vi "Read Dataset and All Attributes (Variant).vi"(4 "Data":variant, 8 "error in (no error)":errorcluster, 10 "Dataset Path":string, 11 "HDF5 Ref":T1) -> (0 "error out":errorcluster, 1 "Data out":variant, 3 "HDF5 Ref out":T1, 5 "Attribute Values":variant[](array[variant]), 7 "Attribute Names":string[](array[string]))   [LabVIEW 2017]
doc: "Reads a dataset and some or all of its attributes."
uses:
  <vilib>/UPVI/lvhdf5/library.llb/HDF5 Ref.ctl
panel:
  # "LVHDF5 Toolkit\nCopyright (c) 2005-2013 by Jason D. Sommerville\nCopyright (c) 2014 by UPVI, LLC.\n\nThis use and distribution of this file is governed by the terms found in \nLICENSE.txt distributed with this toolkit and installed at\n <user.lib>\\_lvhdf5\\LICENSE.txt"
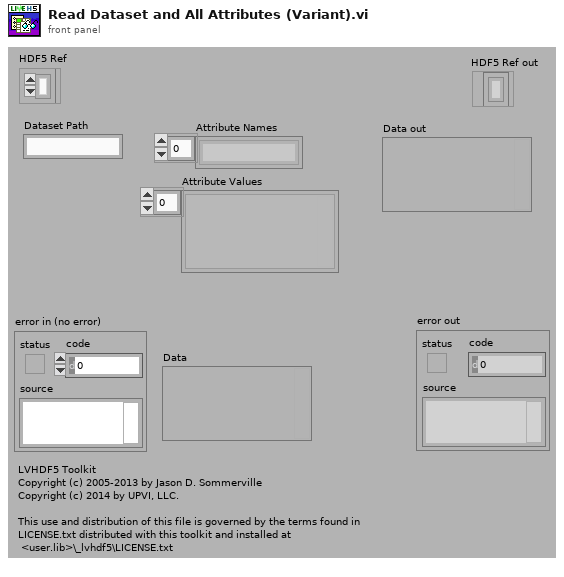
[diagram p1: front panel]
types:
  T1 = typedef "HDF5 Ref.ctl" = refnum<k1>
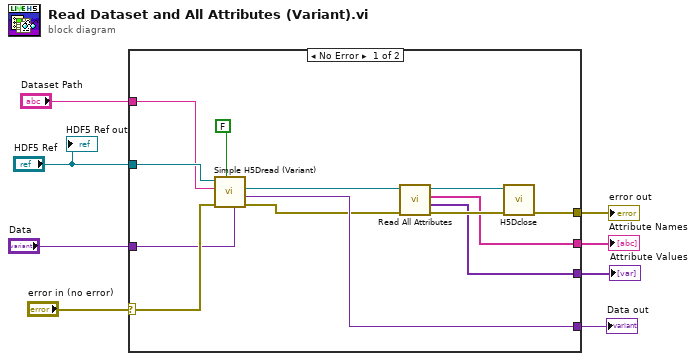
[diagram p0: block diagram]
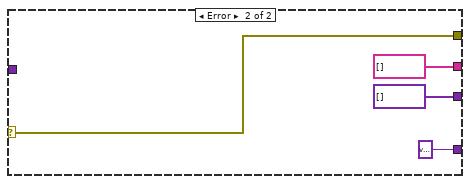
[diagram p2: hidden frame]
diagram:
  n1 = case shown="No Error" "error in (no error)" {
    selector: "error in (no error)" -> [w20 w25]
    tunnel: [w19 w25] -> w7
    tunnel: "HDF5 Ref" -> [w21 _]
    tunnel: [w14 variant ("Data")] -> w5
    tunnel: [w16 string[] [] ("Names")] -> w4
    tunnel: [w15 variant[] [] ("Values")] -> w3
    tunnel: "Dataset Path" -> [w10 _]
    tunnel: "Data" -> [w9 _]
    frame No Error {
      n2 = call <vilib>:"Simple H5Dread (Variant).vi"("Data"=w9, "Close dataset (T)"=FALSE, "error in (no error)"=w20, "Dataset Path"=w10, "HDF5 Ref"=w21) -> ("error out"=w13:errorcluster, "Data out"=w14:variant, "HDF5 Dataset Ref"=w11:T1)  [unwired: 3 in, 1 out]
      n3 = call <vilib>:"Read All Attributes.vi"("error in (no error)"=w13, "HDF5 Ref"=w11) -> ("error out"=w17:errorcluster, "Values"=w15:variant[], "Names"=w16:string[], "HDF5 Ref out"=w18:T1)  [unwired: 4 in]
      n4 = call <vilib>:"H5Dclose.vi"("error in (no error)"=w17, "HDF5 Dataset Ref"=w18) -> ("error out"=w19:errorcluster)  [unwired: 7 in]
    }
    frame Error {
    }
  }
  "error out" <- w7
  "Data out" <- w5
  "Attribute Names" <- w4
  "Attribute Values" <- w3
  "HDF5 Ref out" <- "HDF5 Ref"
